vi "View one AP param scada.vi"(5 "Sensors refs":refnum<vi>[](array[refnum]), 6 "OPC UA.Client refnum":T1, 7 "conninfo":T3={"host"="localhost", "port"="5432", "client_encoding"="WIN1251", "dbname"="system", "user"="postgres", "password"=""}, 8 "error in (no error)":errorcluster, 9 "AIParameters":string[](array[string]), 10 "AI_State":T2[](array[typedef]), 11 "AITable":dbl[](array[numeric]) format="%#.0f") -> (0 "error out":errorcluster)   [LabVIEW 2019, in "Inputs.lvlib"]
uses:
  Database/ctl/Coninfo.ctl
  Ctl/Parameter State.ctl
  <vilib>/OPCUA/controls/OPC UA Client Refnum.ctl
  Ctl/View one AI param State.ctl
  <vilib>/Utility/miscctls.llb/LVRowAndColumnUnsignedTypeDef.ctl
  Ctl/AIParamColumns.ctl
  <vilib>/OPCUA/controls/NodeId.ctl
  Database/select_initial.vi
  Database/PostgreSQL2LabVIEW/libpqUtility/src/PQconnect.vi
  Database/PostgreSQL2LabVIEW/libpqUtility/src/PQclose.vi
  Database/PostgreSQL2LabVIEW/libpqlv/src/PQfinish.vi
  Database/PostgreSQL2LabVIEW/libpqlv/src/PQconnectdb.vi
  Database/PostgreSQL2LabVIEW/libpqlv/src/PQerrorMessage.vi
  Database/PostgreSQL2LabVIEW/libpqlv/src/PQstatus.vi
  <vilib>/dlg_ctls.llb/Space Constant.vi
  Database/PostgreSQL2LabVIEW/libpqUtility/src/PQgetTable.vi
  Database/Progress.vi
  <vilib>/OPCUA/client/Multiple Write Variant.vi
  Inputs.lvlib
  <vilib>/OPCUA/NI OPC UA Client.lvlib
  OPC/OPC addons.lvlib
  Database/PostgreSQL.lvlib
panel:
  in  "sensor num":i32
  in  "instrument_min_offset":dbl min=-32768.0 max=65535.0 step=1.0 format="%#.0f"
  in  "time_const":dbl min=-32768.0 max=65535.0 step=1.0 format="%#.0f"
  in  "instrument_offset":dbl min=-32768.0 max=65535.0 step=1.0 format="%#.0f"
  in  "instrument_gain":dbl min=-32768.0 max=65535.0 step=1.0 format="%#.0f"
  in  "fcode_full":string="кгс/см2"
  out "AI_1":dbl format="%#.1f"
  in  "Param":i32(listbox) caption="Параметры"
  in  "d":dbl min=-32768.0 max=65535.0 step=1.0 format="%#.0f"
  in  "instrument_max_offset":dbl min=-32768.0 max=65535.0 step=1.0 format="%#.0f"
  in  "input_pv_max":dbl format="%#.1f"
  in  "input_pv_min":dbl format="%#.1f"
  in  "input_register_max":dbl min=-32768.0 max=65535.0 step=1.0 format="%#.0f"
  in  "input_register_min":dbl min=-32768.0 max=65535.0 step=1.0 format="%#.0f"
  out "units":string="кгс/см2"
  in  "instrument_range_max":dbl format="%#.1f"
  in  "process_range_max":dbl format="%#.1f"
  in  "process_high_acd":dbl format="%#.1f"
  in  "process_high_alr":dbl format="%#.1f"
  in  "process_low_alr":dbl format="%#.1f"
  in  "process_low_acd":dbl format="%#.1f"
  in  "process_range_min":dbl format="%#.1f"
  in  "instrument_range_min":dbl format="%#.1f"
  # "Настройка пределов"
  # "верхнийний предел параметра"
  # "верхний предел достоверных показаний"
  # "верхний аварийный предел"
  # "верхний предупредительный предел"
  # "нижний предупредительный предел"
  # "нижний аварийный предел"
  # "нижний предел достоверных показаний"
  # "нижний предел параметра"
  # "Настройка смещения и массштабирования параметра"
  # "Y"
  # "массштабирование"
  # "смещение"
  # "X"
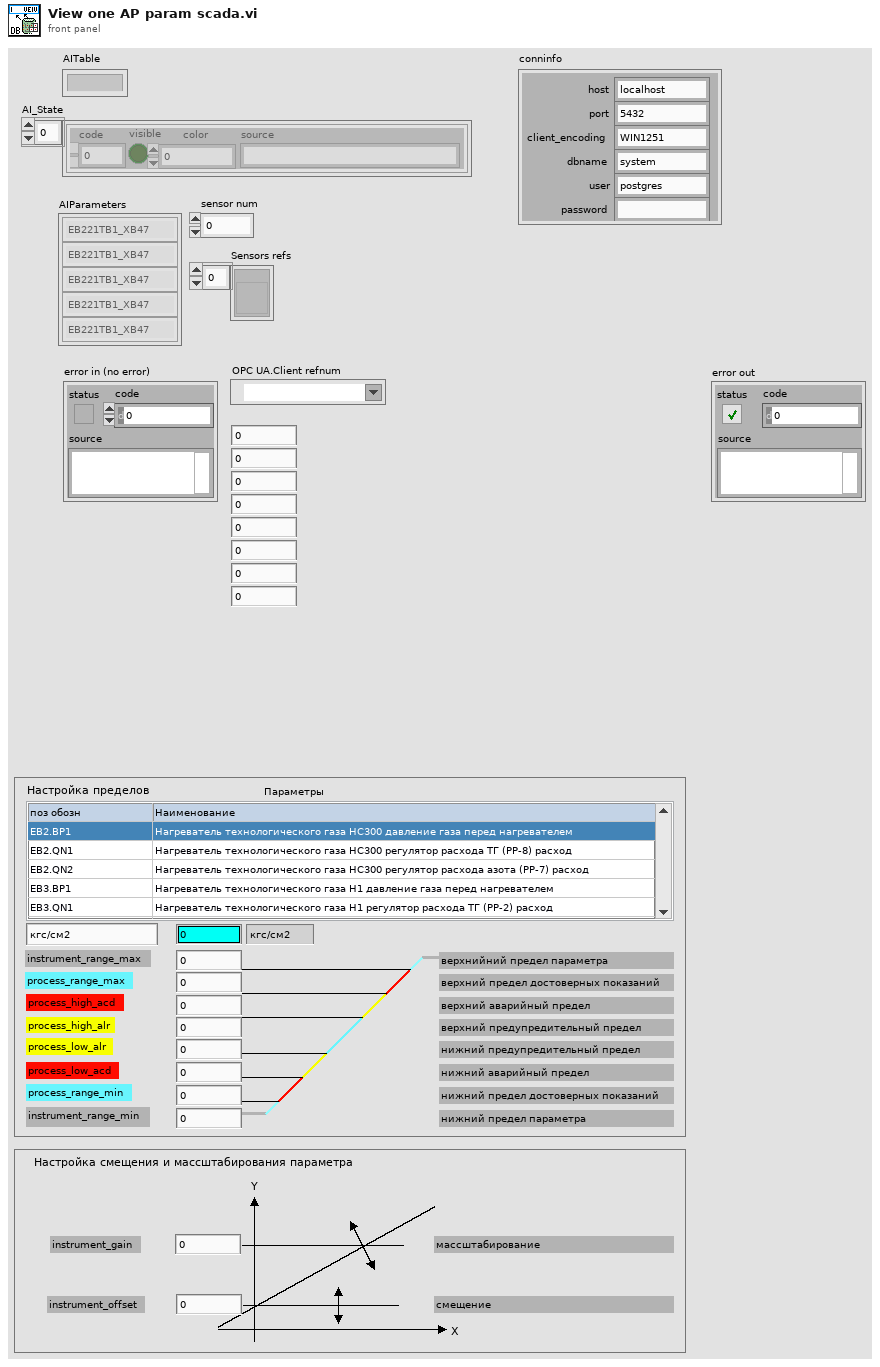
[diagram p1: front panel]
types:
  T1 = typedef "OPC UA Client Refnum.ctl" = refnum<k21>
  T2 = typedef "Inputs.lvlib/Parameter State.ctl" = cluster{"code":i32, "visible":bool, "color":u32, "source":string}
  T3 = typedef "PostgreSQL.lvlib/Coninfo.ctl" = cluster{"host":string, "port":string, "client_encoding":string, "dbname":string, "user":string, "password":string}
  T4 = typedef "Inputs.lvlib/View one AI param State.ctl" = enum16{"init", "change sensor", "wait changes", "write parameters"}
  T5 = typedef "LVRowAndColumnUnsignedTypeDef.ctl" = cluster{"Row":u32, "Column":u32}
  T6 = typedef "NodeId.ctl" = string
  T7 = typedef "Inputs.lvlib/AIParamColumns.ctl" = enum16{"instrument_gain", "instrument_offset", "time_const", "instrument_min_offset", "instrument_range_min", "process_range_min", "process_low_acd", "process_low_alr", "process_high_alr", "process_high_acd", "process_range_max", "instrument_range_max", "instrument_max_offset", "d", "input_register_min", "input_register_max", "input_pv_min", "input_pv_max", "module_fcode_full", "control_channel_num", "ip_adress", "fcode", "fcodef", "fcode_full", "fname", "process_units"}
  T8 = typedef "Write Variant Request.ctl" = cluster{"node ID":T6, "value":variant, "timestamp (current time)":timestamp, "node status":T9}
  T9 = typedef "Write Status.ctl" = u32
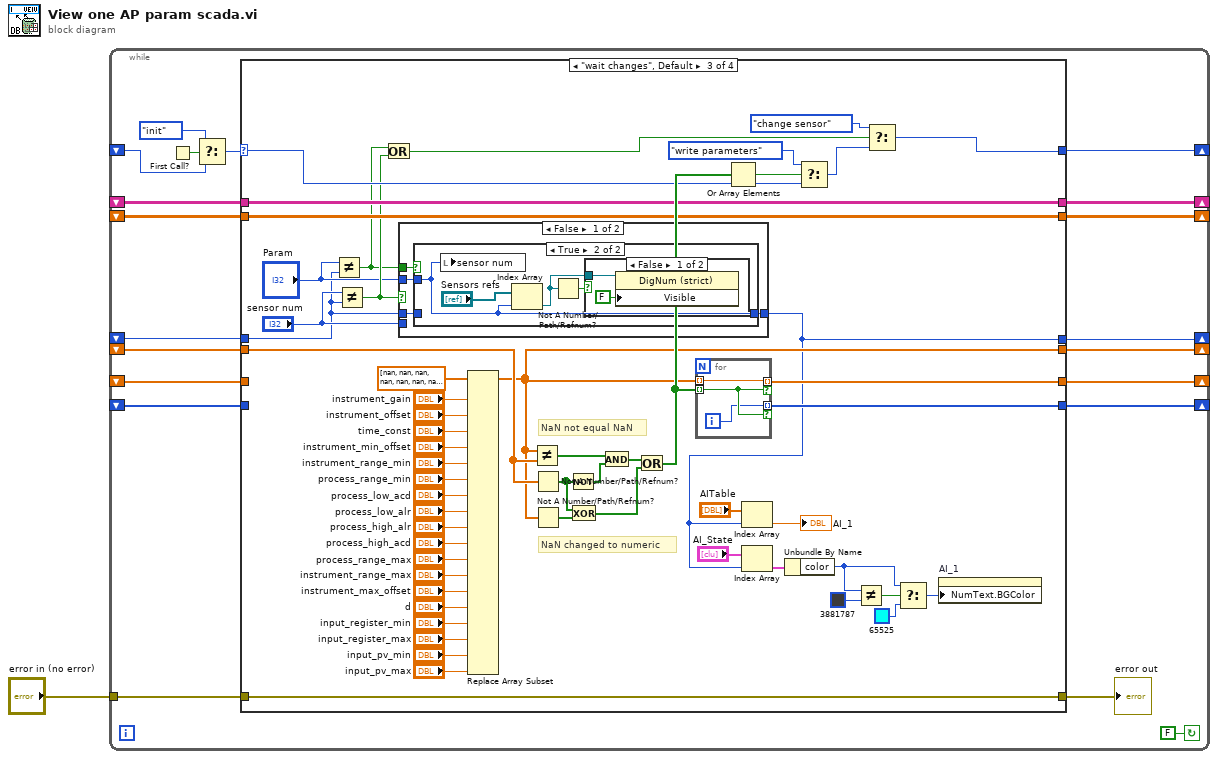
[diagram p0: block diagram]
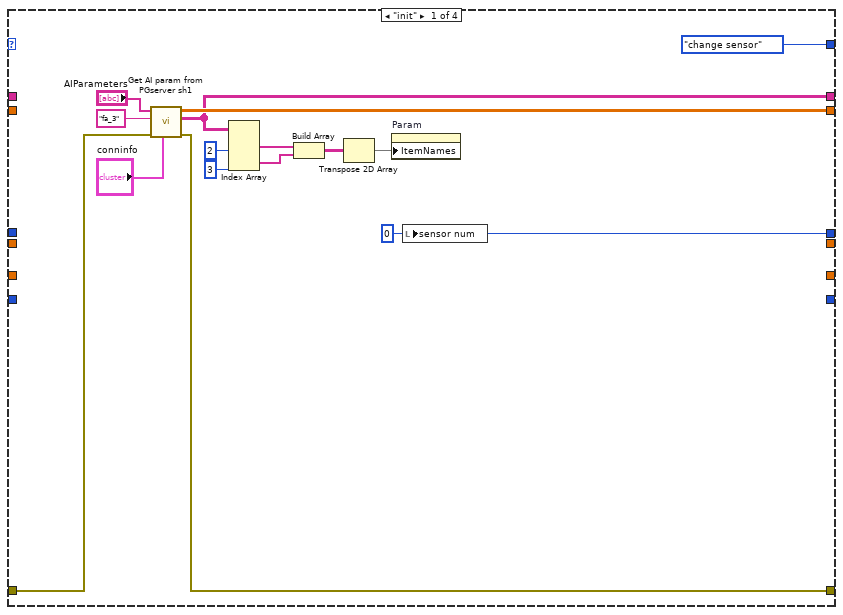
[diagram p2: hidden frame]
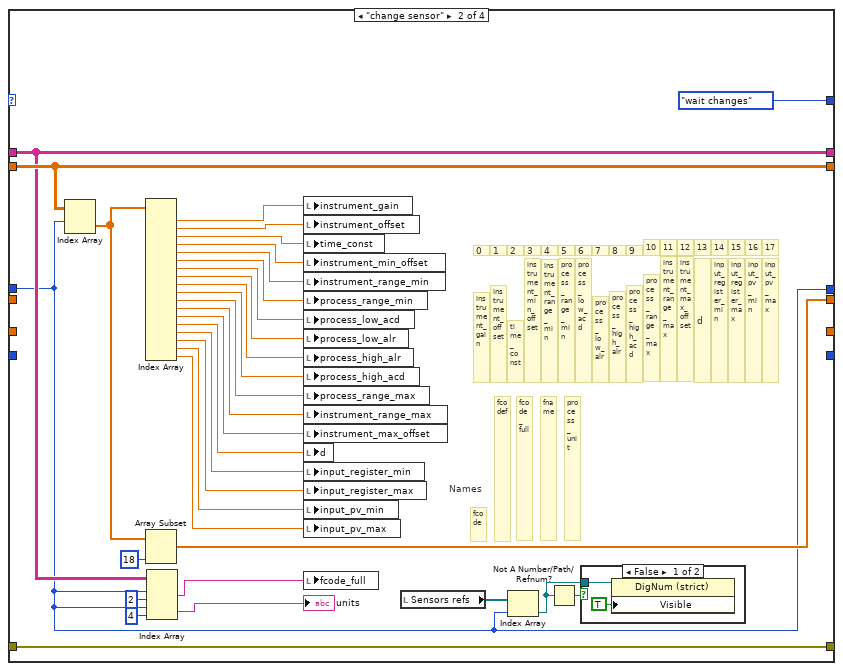
[diagram p3: hidden frame]
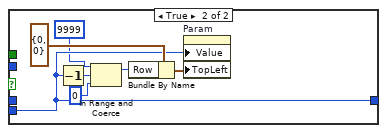
[diagram p7: hidden frame]
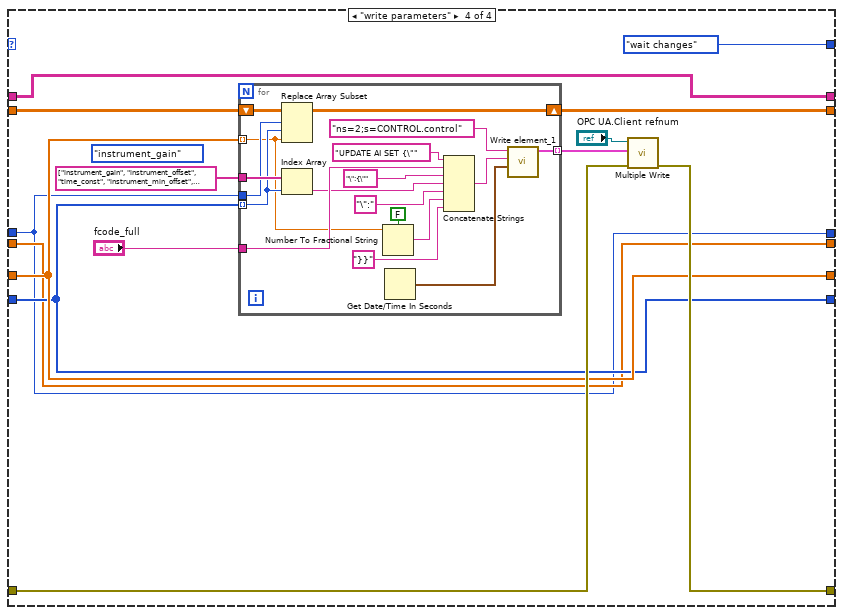
[diagram p8: hidden frame]
diagram:
  n1 = while {
    shift-right: [w19] -> _
    shift-left: _ -> [w17]
    shift-right: [w18] -> _
    shift-left: _ -> [w16]
    shift-right: [w15] -> _
    shift-left: _ -> [w14]
    tunnel: "error in (no error)" -> [w13]
    shift-right: [w12] -> _
    shift-left: _ -> [w4]
    shift-right: [w11] -> _
    shift-left: _ -> [w9]
    shift-right: [w10] -> _
    shift-left: _ -> [w8]
    shift-right: [w7] -> _
    shift-left: _ -> [w6]
    stop <- FALSE ("Boolean") continue-if-true
    n2 = First Call?() -> (First Call?: T/F=w5:bool)
    n3 = Select(t=View_one_AI_param_State."init", s=w5, f=w4) -> (s? t:f=w2:T4)
    n4 = case shown="\"wait changes\", Default" w2 {
      selector: w2 -> [_ _ w87 _]
      tunnel: w6 -> [_ w38 w78 w148]
      tunnel: w16 -> [_ w51 w98 w158]
      tunnel: w17 -> [_ w52 w93 w160]
      tunnel: [w29 w42 w90 w161] -> w21
      tunnel: [_ w50 w104 w149] -> w15
      tunnel: w14 -> [_ _ w107 w149]
      tunnel: [w31 w52 w93 w159] -> w19
      tunnel: [w28 w51 w98 w158] -> w18
      tunnel: w13 -> [w30 w42 w90 w157]
      tunnel: [View_one_AI_param_State."change sensor" View_one_AI_param_State."wait changes" w86 View_one_AI_param_State."wait changes"] -> w12
      tunnel: [_ _ w92 w151] -> w11
      tunnel: [_ _ w91 w150] -> w10
      tunnel: w9 -> [_ _ _ w151]
      tunnel: w8 -> [_ _ _ w150]
      tunnel: [w22 w38 w77 w148] -> w7
      frame "init" {
        w22 = 0 ("sensor num")
        n5 = call "Get AI param from PGserver sh1.vi"("conninfo"="conninfo", "error in (no error)"=w30, "AIParamTable"="fa_3", "AIParameters"="AIParameters") -> ("error out"=w29:errorcluster, "Names table"=w28:string[][], "Parameters table"=w31:dbl[][])  [unwired: 5 in]
        n6 = Index Array(array=w28, index (col) #1=2 ("index (row)"), index (col) #2=3 ("index (row)")) -> (element #1=w26:string[], element #2=w25:string[])  [unwired: 2 in]
        n7 = Build Array(w26, w25) -> (w24:string[][])
        n8 = Transpose 2D Array(2D array=w24) -> (transposed array=w23:string[][])
        n9 = property on="Param" class="MCListbox (strict)"("ItemNames"=w23) -> ()  [unwired: 2 in, 2 out]
        n10 = local write "sensor num"(w22) -> ()
      }
      frame "change sensor" {
        # "fcodef"
        # "process_unit"
        # "fname"
        # "fcode_full"
        # "fcode"
        # "Names"
        # "input_pv_max"
        # "input_pv_min"
        # "input_register_max"
        # "input_register_min"
        # "d"
        # "instrument_max_offset"
        # "instrument_range_max"
        # "process_range_max"
        # "process_high_acd"
        # "process_high_alr"
        # "process_low_alr"
        # "process_low_acd"
        # "process_range_min"
        # "instrument_range_min"
        # "instrument_min_offset"
        # "time_const"
        # "instrument_gain"
        # "instrument_offset"
        # "17"
        # "16"
        # "15"
        # "14"
        # "13"
        # "12"
        # "11"
        # "10"
        # "9"
        # "8"
        # "7"
        # "6"
        # "5"
        # "4"
        # "3"
        # "2"
        # "0"
        # "1"
        n11 = Index Array(array=w52, index (row)=w38) -> (element=w54:dbl[])  [unwired: 1 in]
        n12 = Index Array(array=w54) -> (element #1=w44:dbl, element #2=w45:dbl, element #3=w46:dbl, element #4=w47:dbl, element #5=w68:dbl, element #6=w67:dbl, element #7=w66:dbl, element #8=w65:dbl, element #9=w64:dbl, element #10=w63:dbl, element #11=w62:dbl, element #12=w61:dbl, element #13=w56:dbl, element #14=w55:dbl, element #15=w60:dbl, element #16=w59:dbl, element #17=w58:dbl, element #18=w57:dbl)  [unwired: 18 in]
        n13 = Array Subset(array=w54, length=18) -> (w50:dbl[])  [unwired: 1 in]
        n14 = Index Array(array=w51, index (row) #1=w38, index (col) #1=2 ("length"), index (row) #2=w38, index (col) #2=4 ("length")) -> (element #1=w43:string, element #2=→"units":string)
        n15 = local write "instrument_gain"(w44) -> ()
        n16 = local write "instrument_offset"(w45) -> ()
        n17 = local write "time_const"(w46) -> ()
        n18 = local write "instrument_min_offset"(w47) -> ()
        n19 = local write "instrument_range_min"(w68) -> ()
        n20 = local write "process_range_min"(w67) -> ()
        n21 = local write "process_low_acd"(w66) -> ()
        n22 = local write "process_low_alr"(w65) -> ()
        n23 = local write "process_high_alr"(w64) -> ()
        n24 = local write "process_high_acd"(w63) -> ()
        n25 = local write "process_range_max"(w62) -> ()
        n26 = local write "instrument_range_max"(w61) -> ()
        n27 = local write "instrument_max_offset"(w56) -> ()
        n28 = local write "d"(w55) -> ()
        n29 = local write "input_register_min"(w60) -> ()
        n30 = local write "input_register_max"(w59) -> ()
        n31 = local write "input_pv_min"(w58) -> ()
        n32 = local write "input_pv_max"(w57) -> ()
        n33 = local write "fcode_full"(w43) -> ()
        n34 = local read "Sensors refs"() -> (w37:refnum<vi>[])
        n35 = Index Array(array=w37, index=w38) -> (element=w39:refnum<vi>)
        n36 = Not A Number/Path/Refnum?(number/path/refnum=w39) -> (NaN/Path/Refnum?=w40:bool)
        n37 = case shown="False" w40 {
          tunnel: w39 -> [w71 _]
          frame False {
            n38 = property on="Property Node" class="DigNum (strict)"(reference=w71, "Visible"=TRUE ("Blinking")) -> ()  [unwired: 1 in, 2 out]
          }
          frame True {
          }
        }
      }
      frame "wait changes", Default {
        # "NaN changed to numeric"
        # "NaN not equal NaN"
        n39 = Not Equal?(x="Param", y=w78) -> (x != y?=w81:bool)
        n40 = Not Equal?(x="sensor num", y=w78) -> (x != y?=w83:bool)
        n41 = Or(x=w81, y=w83) -> (x .or. y?=w82:bool)
        n42 = case shown="False" w83 {
          tunnel: "sensor num" -> [_ w140]
          tunnel: w81 -> [w130 _]
          tunnel: [w128 w140] -> w77
          tunnel: "Param" -> [w129 _]
          tunnel: w78 -> [w127 _]
          frame False {
            n43 = case shown="True" w130 {
              tunnel: w129 -> [_ w134]
              tunnel: [w131 w134] -> w128
              tunnel: w127 -> [w131 _]
              frame False {
              }
              frame True {
                n44 = local write "sensor num"(w134) -> ()
                n45 = Index Array(array="Sensors refs", index=w134) -> (element=w132:refnum<vi>)
                n46 = Not A Number/Path/Refnum?(number/path/refnum=w132) -> (NaN/Path/Refnum?=w133:bool)
                n47 = case shown="False" w133 {
                  tunnel: w132 -> [w137 _]
                  frame False {
                    n48 = property on="Property Node" class="DigNum (strict)"(reference=w137, "Visible"=FALSE ("Blinking")) -> ()  [unwired: 1 in, 2 out]
                  }
                  frame True {
                  }
                }
              }
            }
          }
          frame True {
            n49 = Decrement(x=w140) -> (x-1=w141:i32)
            n50 = In Range and Coerce(upper limit=9999, x=w141, lower limit=0) -> (coerced(x)=w142:i32)  [unwired: 1 out]
            n51 = Bundle By Name(cluster=T5 {"Row"=0, "Column"=0} ("Top Left Visible Cell"), "Row"=w142) -> (w143:T5)
            n52 = property on="Param" class="MCListbox (strict)"("Value"=w140, "TopLeft"=w143) -> ()  [unwired: 2 in, 2 out]
          }
        }
        n53 = Replace Array Subset(array=dbl[] [nan, nan, nan, nan, nan, nan, nan, nan, nan, nan, nan, nan, nan, nan, nan, nan, nan, nan] ("Parameters table"), new element #1="instrument_gain", new element #2="instrument_offset", new element #3="time_const", new element #4="instrument_min_offset", new element #5="instrument_range_min", new element #6="process_range_min", new element #7="process_low_acd", new element #8="process_low_alr", new element #9="process_high_alr", new element #10="process_high_acd", new element #11="process_range_max", new element #12="instrument_range_max", new element #13="instrument_max_offset", new element #14="d", new element #15="input_register_min", new element #16="input_register_max", new element #17="input_pv_min", new element #18="input_pv_max") -> (w104:dbl[])  [unwired: 18 in]
        n54 = Not Equal?(x=w104, y=w107) -> (x != y?=w105:bool[])
        n55 = Not A Number/Path/Refnum?(number/path/refnum=w107) -> (NaN/Path/Refnum?=w100:bool[])
        n56 = Not A Number/Path/Refnum?(number/path/refnum=w104) -> (NaN/Path/Refnum?=w99:bool[])
        n57 = Not(x=w100) -> (.not. x?=w101:bool[])
        n58 = Exclusive Or(1:w99, 2:w100) -> (0:w103:bool[])
        n59 = And(x=w105, y=w101) -> (x .and. y?=w102:bool[])
        n60 = Or(x=w102, y=w103) -> (x .or. y?=w106:bool[])
        n61 = for {
          tunnel: w104 -> [w147] mode=indexing
          tunnel: w106 -> [w146] mode=indexing
          tunnel: [w147] -> w92 mode=indexing if=w146
          tunnel: [w145] -> w91 mode=indexing if=w146
          i -> [w145]
        }
        n62 = Or Array Elements(Boolean array=w106) -> (logical OR=w88:bool)
        n63 = Index Array(array="AITable", index=w77) -> (element=→"AI_1":dbl)
        n64 = Index Array(array="AI_State", index=w77) -> (element=w108:T2)
        n65 = Unbundle By Name(w108) -> ("color"=w74:u32)
        n66 = Select(t=View_one_AI_param_State."write parameters", s=w88, f=w87) -> (s? t:f=w85:T4)
        n67 = Not Equal?(x=w74, y=u32 3881787 ("color")) -> (x != y?=w75:bool)
        n68 = Select(t=View_one_AI_param_State."change sensor", s=w82, f=w85) -> (s? t:f=w86:T4)
        n69 = Select(t=w74, s=w75, f=u32 65525 ("color")) -> (s? t:f=w73:u32)
        n70 = property on="AI_1" class="DigNum (strict)"("NumText.BGColor"=w73) -> ()  [unwired: 2 in, 2 out]
      }
      frame "write parameters" {
        (unwired) AIParamColumns."instrument_gain" ("AIParamColumns")
        n71 = for {
          tunnel: w148 -> [w176]
          tunnel: string[] ["instrument_gain", "instrument_offset", "time_const", "instrument_min_offset", "instrument_range_min", "process_range_min", "process_low_acd", "process_low_alr", "process_high_alr", "process_high_acd", "process_range_max", "instrument_range_max", "instrument_max_offset", "d", "input_register_min", "input_register_max", "input_pv_min", "input_pv_max", "fcode", "fcodef", "fcode_full", "fname", "process_units"] ("AIParamColumns") -> [w179]
          tunnel: w150 -> [w173] mode=indexing
          tunnel: w151 -> [w164] mode=indexing
          shift-right: [w177] -> w159
          shift-left: w160 -> [w178]
          tunnel: "fcode_full" -> [w166]
          tunnel: [w162] -> w154 mode=indexing
          n72 = Replace Array Subset(array=w178, new element=w164, index (row)=w176, index (col)=w173) -> (w177:dbl[][])
          n73 = Index Array(array=w179, index=w173) -> (element=w165:string)
          n74 = Number To Fractional String(use system decimal point (T)=FALSE, number=w164) -> (F-format string=w172:string)  [unwired: 2 in]
          n75 = Get Date/Time In Seconds() -> (seconds since 1Jan1904=w174:timestamp)
          n76 = Concatenate Strings("UPDATE AI SET {\"" ("string"), w166, "\":{\"" ("string"), w165, "\":" ("string"), w172, "}}" ("string")) -> (w163:string)
          n77 = call "Write element_1.vi"("seconds since 1Jan1904"=w174, "Variant"=w163, "node ID"=T6 "ns=2;s=CONTROL.control") -> ("request out"=w162:T8)  [unwired: 8 in]
        }
        n78 = call-poly <vilib>:"Multiple Write.vi"("error in (no error)"=w157, "requests"=w154, "OPC UA client refnum in"="OPC UA.Client refnum") -> ("error out"=w161:errorcluster)  [unwired: 5 in, 3 out]
      }
    }
    "error out" <- w21
  }
